vi "Get FPGA Resource Name.vi"(8 "error in (no error)":errorcluster, 10 "RIO (0)":u8, 11 "IP address":string) -> (0 "error out":errorcluster, 3 "resource name":string)   [LabVIEW 2017, in "NI_Robotics_Starter Kit Host_FPGA.lvclass"]
uses:
  <vilib>/robotics/Starter Kit/FPGA Host Interface/NI_Robotics_Starter Kit Host_FPGA.lvclass
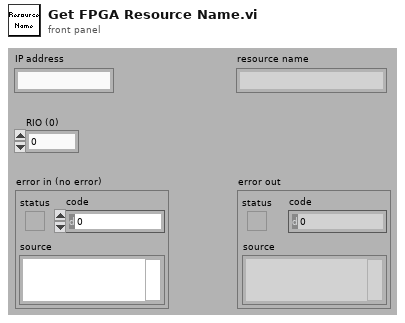
[diagram p1: front panel]
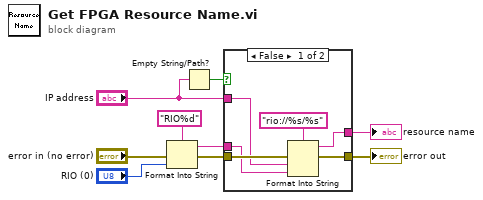
[diagram p0: block diagram]
diagram:
  n1 = Format Into String(format string="RIO%d", error in="error in (no error)", "RIO (0)") -> (resulting string=w3:string, error out=w4:errorcluster)  [unwired: 1 in]
  n2 = Empty String/Path?(string/path="IP address") -> (empty?=w9:bool)
  n3 = case shown="False" w9 {
    tunnel: w4 -> [w15 w17]
    tunnel: "IP address" -> [w13 _]
    tunnel: [w14 w17] -> w6
    tunnel: w3 -> [w12 w16]
    tunnel: [w11 w16] -> w7
    frame False {
      n4 = Format Into String(format string="rio://%s/%s", error in=w15, w13, w12) -> (resulting string=w11:string, error out=w14:errorcluster)  [unwired: 1 in]
    }
    frame True {
    }
  }
  "error out" <- w6
  "resource name" <- w7
